vi "Stop Core.vi"(10 "final error code":i32, 11 "LeftListboxViewManager in":refnum<class "LeftListboxViewManager.lvclass">) -> (3 "LeftListboxViewManager out":refnum<class "LeftListboxViewManager.lvclass">)   [LabVIEW 2020, in "LeftListboxViewManager.lvlib" / "LeftListboxViewManager.lvclass"]
doc: "(<B>Filename</B>: Actor Framework.lvlib:Actor.lvclass:Stop Core.vi)\n\nDefines what the actor does before it stops. Use the <B>final error code</B> input to determine whether the actor shut down in response to an error.\n\nBy default, this method does nothing. A descendant class may override it to define behavior, such as shutting down any processes the actor initiated in its override of the Actor Core method.\n\n<License>\nCopyright © 2017 Composed Systems, LLC | All rights reserved\nwww.composed.io\n\nAuthor: Ethan Stern <ethan.stern@composed.io>\n\nThis software is provided \"AS IS\" WITHOUT WARRANTIES, either express or implied, AND IS FOR EDUCATIONAL PURPOSES ONLY.\n</License>"
uses:
  <vilib>/gpm_packages/@cs/ViewManager/source/LeftListboxViewManager/LeftListboxViewManager.lvclass
  <vilib>/gpm_packages/@cs/ViewManager/source/LeftListboxViewManager/LeftListboxViewManager.lvclass/LeftListboxViewManager.ctl
  <vilib>/gpm_packages/@cs/mva-viewable/Source/IViewManager/IViewManager/IViewManager.lvclass
  <vilib>/gpm_packages/@cs/mva-viewable/Source/IViewable/ProtectedSubpanel/ProtectedSubpanel.lvclass
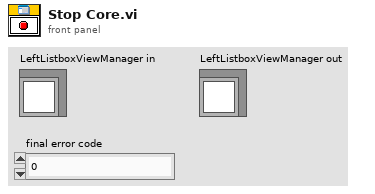
[diagram p1: front panel]
types:
  T1 = typedef "IViewable.lvlib/ProtectedSubpanel.lvclass/Protected Subpanel Reference.ctl" = refnum<data-value>
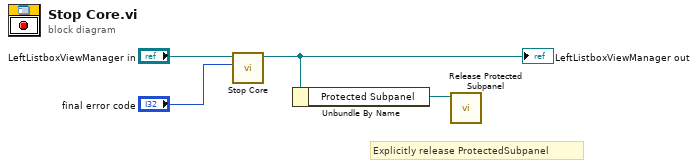
[diagram p0: block diagram]
diagram:
  # "Explicitly release ProtectedSubpanel"
  n1 = call-parent "Stop Core.vi"("final error code"="final error code", "IViewManager in"="LeftListboxViewManager in") -> ("IViewManager out"=w2:refnum<class "LeftListboxViewManager.lvclass">)  [unwired: 9 in]
  "LeftListboxViewManager out" <- w2
  n2 = Unbundle By Name(w2) -> ("Protected Subpanel"=w1:T1)
  n3 = call <vilib>:"Release Protected Subpanel.vi"("Protected Subpanel"=w1) -> ()  [unwired: 10 in, 1 out]
